vi "Clap Logic.vi"(8 "error in (no error)":errorcluster, 9 "Clapper Out":bool, 10 "Clapper In":bool, 11 "Clap State":T1) -> (0 "error out":errorcluster, 3 "Clap State":T1)   [LabVIEW 2014]
doc: "Swings the clapper in / out one state based on Teleop input.\nStates wrap around, so moving out past Out will swing the clapper all the way In, and vice versa."
uses:
  Arm clapper state.ctl
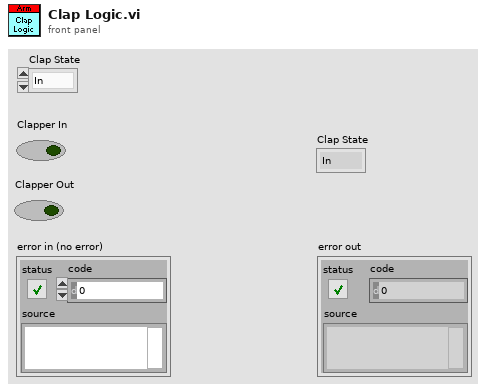
[diagram p1: front panel]
types:
  T1 = typedef "Arm clapper state.ctl" = enum16{"In", "Tote Closed", "Bin Closed", "Straight", "Open"}
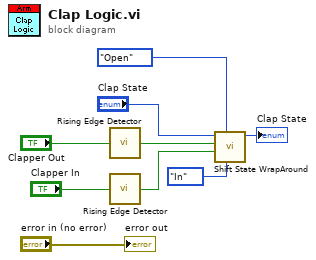
[diagram p0: block diagram]
diagram:
  n1 = call "Rising Edge Detector.vi"("Input"="Clapper Out") -> ("Rising edge?"=w4:bool)
  n2 = call "Rising Edge Detector.vi"("Input"="Clapper In") -> ("Rising edge?"=w3:bool)
  n3 = call "Shift State WrapAround.vi"("Lower bound"=Arm_clapper_state."In" ("Clap State"), "Upper bound"=Arm_clapper_state."Open" ("Clap State"), "Decrement"=w3, "Increment"=w4, "State in"="Clap State") -> ("State out"=→"Clap State":i32)  [unwired: 6 in]
  "error out" <- "error in (no error)"
